vi "NewQuestionTableName(SubVI).vi"(9 "For Tree Control":dbl, 11 "connection reference":T1) -> (1 "For Tree Control":string, 3 "String":string)   [LabVIEW 2013]
uses:
  <vilib>/addons/database/Connection.llb/Conn ObjectReference.ctl
  FYP_LabviewGlobal(SubVI).vi
  <vilib>/addons/database/NI_Database_API.lvlib
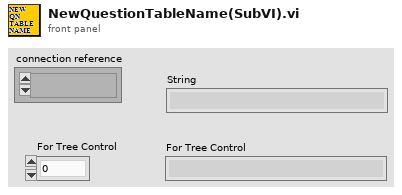
[diagram p1: front panel]
types:
  T1 = typedef "NI_Database_API.lvlib/Conn ObjectReference.ctl" = refnum<k1>
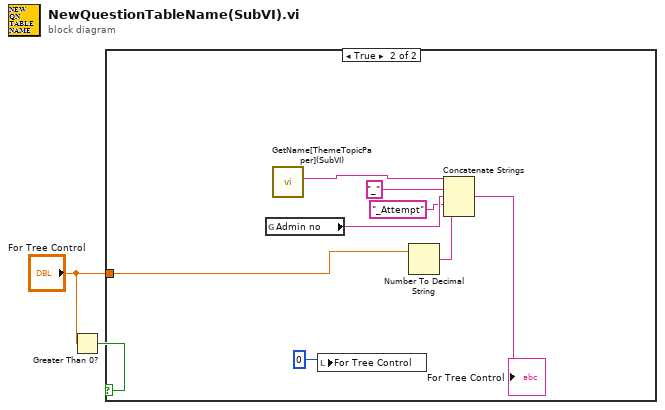
[diagram p0: block diagram]
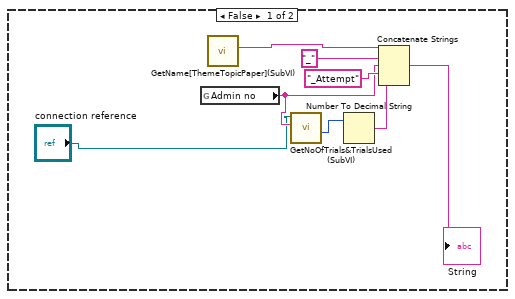
[diagram p2: hidden frame]
diagram:
  n1 = Greater Than 0?(x="For Tree Control") -> (x > 0?=w1:bool)
  n2 = case shown="True" w1 {
    tunnel: "For Tree Control" -> [_ w12]
    frame False {
      n3 = global read "FYP_LabviewGlobal(SubVI).vi" "Admin no"() -> (w4:string)
      n4 = call "GetName[ThemeTopicPaper](SubVI).vi"() -> ("Path for Score Table"=w8:string)  [unwired: 11 in]
      n5 = call "GetNoOfTrials&TrialsUsed(SubVI).vi"("Admin no"=w4, "Refnum in"="connection reference") -> ("NoOfTrialsUsed"=w10:i32)  [unwired: 8 in, 1 out]
      n6 = Number To Decimal String(number=w10) -> (decimal integer string=w5:string)  [unwired: 1 in]
      n7 = Concatenate Strings(w8, "_", w4, "_Attempt", w5) -> (→"String":string)
    }
    frame True {
      n8 = global read "FYP_LabviewGlobal(SubVI).vi" "Admin no"() -> (w18:string)
      n9 = call "GetName[ThemeTopicPaper](SubVI).vi"() -> ("Path for Score Table"=w14:string)  [unwired: 11 in]
      n10 = local write "For Tree Control"(0) -> ()
      n11 = Number To Decimal String(number=w12) -> (decimal integer string=w17:string)  [unwired: 1 in]
      n12 = Concatenate Strings(w14, "_", w18, "_Attempt", w17) -> (→"For Tree Control":string)
    }
  }
